vi "Get All Channels.vi"(8 "error in (no error)":errorcluster, 11 "SysDef Ref":T1) -> (0 "error out":errorcluster, 1 "Write Channels":string[](array[string]), 2 "Read Channels":string[](array[string]), 3 "SysDef Ref Out":T1)   [LabVIEW 2024]
uses:
  <userlib>/SimpleSysDef/_SubVIs/System Definition Reference.ctl
  NationalInstruments.VeriStand.SystemDefinitionAPI
  NationalInstruments.VeriStand.SystemStorage
  <userlib>/SimpleSysDef/Simple SysDef API.lvlib
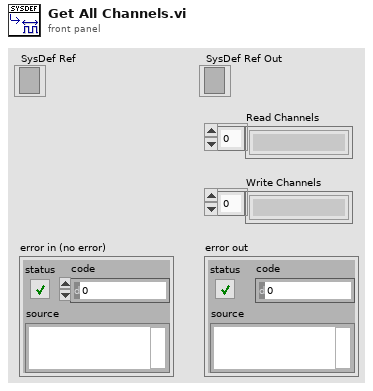
[diagram p1: front panel]
types:
  T1 = typedef "Simple SysDef API.lvlib/System Definition Reference.ctl" = refnum<k24>
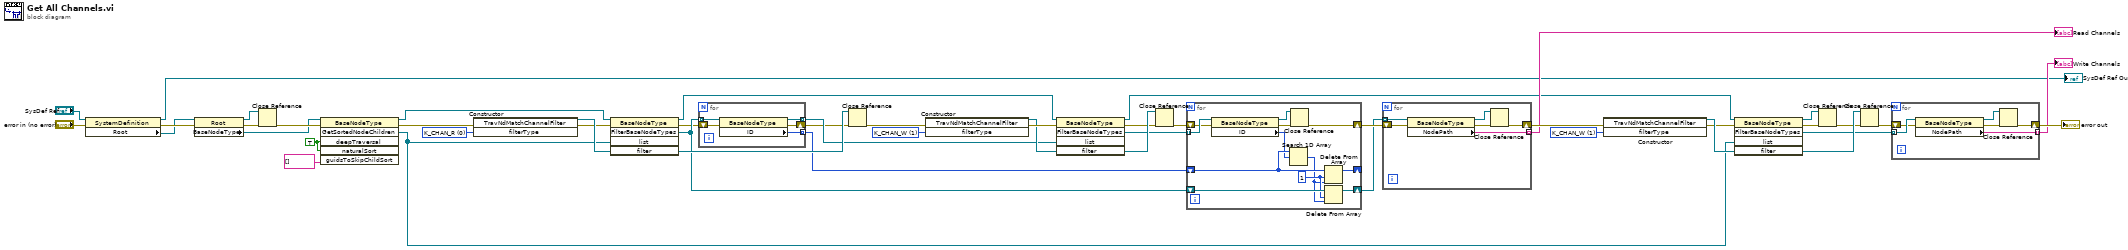
[diagram p0: block diagram]
diagram:
  w16 = u8 1 items=["K_CHAN_R", "K_CHAN_W", "K_CHAN_VOLT", "K_CHAN_FAULT"] ("filterType")
  w25 = TRUE ("deepTraversal")
  w20 = u8 1 items=["K_CHAN_R", "K_CHAN_W", "K_CHAN_VOLT", "K_CHAN_FAULT"] ("filterType")
  w19 = u8 0 items=["K_CHAN_R", "K_CHAN_W", "K_CHAN_VOLT", "K_CHAN_FAULT"] ("filterType")
  n1 = property class="SystemDefinition"(reference="SysDef Ref", error in="error in (no error)") -> (reference out=→"SysDef Ref Out":T1, error out=w18:errorcluster, "Root"=w17:refnum<k24>)
  n2 = property class="Root"(reference=w17, error in=w18) -> (reference out=w32:refnum<k24>, error out=w33:errorcluster, "BaseNodeType"=w23:refnum<k24>)
  n3 = Close Reference(reference=w32, error in (no error)=w33) -> (error out=w38:errorcluster)
  n4 = invoke class="BaseNodeType" method="GetSortedNodeChildren"(reference=w23, error in=w38, "deepTraversal"=w25, "naturalSort"=w25, "guidsToSkipChildSort"=string[] []) -> (reference out=w26:refnum<k24>, error out=w37:errorcluster, "GetSortedNodeChildren"=w29:refnum<k24>[])  [unwired: 1 in, 3 out]
  n5 = constructor class="TravNdMatchChannelFilter"(error in=w37, "filterType"=w19) -> (reference out=w39:refnum<k24>, error out=w36:errorcluster)  [unwired: 2 in, 2 out]
  n6 = invoke class="BaseNodeType" method="FilterBaseNodeTypes"(reference=w26, error in=w36, "list"=w29, "filter"=w39) -> (reference out=w13:refnum<k24>, error out=w2:errorcluster, "FilterBaseNodeTypes"=w4:refnum<k24>[])  [unwired: 1 in, 2 out]
  n7 = for {
    tunnel: w4 -> [w50] mode=indexing
    tunnel: [w49] -> w6 mode=indexing
    tunnel: [w48] -> w3 mode=indexing
    shift-right: [w46] -> w1
    shift-left: w2 -> [w47]
    n8 = property class="BaseNodeType"(reference=w50, error in=w47) -> (reference out=w48:refnum<k24>, error out=w46:errorcluster, "ID"=w49:u64)
  }
  n9 = Close Reference(reference=w39, error in (no error)=w1) -> (error out=w14:errorcluster)
  n10 = constructor class="TravNdMatchChannelFilter"(error in=w14, "filterType"=w16) -> (reference out=w11:refnum<k24>, error out=w15:errorcluster)  [unwired: 2 in, 2 out]
  n11 = invoke class="BaseNodeType" method="FilterBaseNodeTypes"(reference=w13, error in=w15, "list"=w3, "filter"=w11) -> (reference out=w12:refnum<k24>, error out=w10:errorcluster, "FilterBaseNodeTypes"=w7:refnum<k24>[])  [unwired: 1 in, 2 out]
  n12 = Close Reference(reference=w11, error in (no error)=w10) -> (error out=w9:errorcluster)
  n13 = for {
    tunnel: w7 -> [w59] mode=indexing
    shift-right: [w61] -> _
    shift-left: w6 -> [w62]
    shift-right: [w60] -> w8
    shift-left: w9 -> [w58]
    shift-right: [w51] -> w5
    shift-left: w4 -> [w54]
    w53 = 1 ("length")
    n14 = property class="BaseNodeType"(reference=w59, error in=w58) -> (reference out=w56:refnum<k24>, error out=w57:errorcluster, "ID"=w55:u64)
    n15 = Search 1D Array(1D array=w62, element=w55) -> (index of element=w52:i32)  [unwired: 1 in]
    n16 = Close Reference(reference=w56, error in (no error)=w57) -> (error out=w60:errorcluster)
    n17 = Delete From Array(array=w62, length=w53, index=w52) -> (array with subset deleted=w61:u64[])  [unwired: 1 out]
    n18 = Delete From Array(array=w54, length=w53, index=w52) -> (array with subset deleted=w51:refnum<k24>[])  [unwired: 1 out]
  }
  n19 = for {
    tunnel: w5 -> [w68] mode=indexing
    tunnel: [w67] -> w27 mode=indexing
    shift-right: [w64] -> w35
    shift-left: w8 -> [w66]
    n20 = property class="BaseNodeType"(reference=w68, error in=w66) -> (reference out=w63:refnum<k24>, error out=w65:errorcluster, "NodePath"=w67:string)
    n21 = Close Reference(reference=w63, error in (no error)=w65) -> (error out=w64:errorcluster)
  }
  "Read Channels" <- w27
  n22 = constructor class="TravNdMatchChannelFilter"(error in=w35, "filterType"=w20) -> (reference out=w43:refnum<k24>, error out=w34:errorcluster)  [unwired: 2 in, 2 out]
  n23 = invoke class="BaseNodeType" method="FilterBaseNodeTypes"(reference=w12, error in=w34, "list"=w29, "filter"=w43) -> (reference out=w40:refnum<k24>, error out=w41:errorcluster, "FilterBaseNodeTypes"=w28:refnum<k24>[])  [unwired: 1 in, 2 out]
  n24 = Close Reference(reference=w40, error in (no error)=w41) -> (error out=w42:errorcluster)
  n25 = Close Reference(reference=w43, error in (no error)=w42) -> (error out=w44:errorcluster)
  n26 = for {
    tunnel: w28 -> [w74] mode=indexing
    tunnel: [w73] -> w30 mode=indexing
    shift-right: [w70] -> w45
    shift-left: w44 -> [w72]
    n27 = property class="BaseNodeType"(reference=w74, error in=w72) -> (reference out=w69:refnum<k24>, error out=w71:errorcluster, "NodePath"=w73:string)
    n28 = Close Reference(reference=w69, error in (no error)=w71) -> (error out=w70:errorcluster)
  }
  "error out" <- w45
  "Write Channels" <- w30
